vi "Calculate Odd Parity Bit (Array).vi"(0 "Bytes":u8[](array[numeric]) format="%02x", 11 "error in (no error)":errorcluster) -> (4 "Odd Parity Bit":u8, 15 "error out":errorcluster)   [LabVIEW 2018, in "MIPI RFFE API.lvlib"]
uses:
  MIPI RFFE API.lvlib
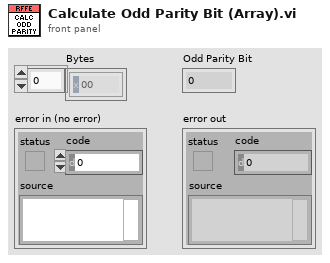
[diagram p1: front panel]
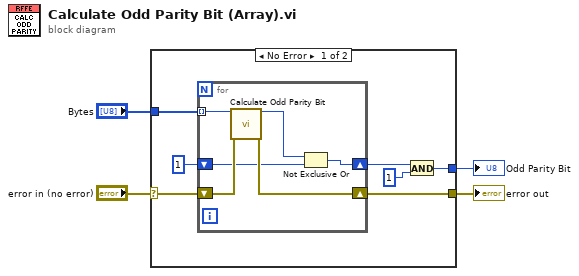
[diagram p0: block diagram]
diagram:
  n1 = case shown="No Error" "error in (no error)" {
    selector: "error in (no error)" -> [w11 w18]
    tunnel: [w10 w18] -> w3
    tunnel: "Bytes" -> [w9 _]
    tunnel: [w6 _] -> w1
    frame No Error {
      n2 = for {
        shift-right: [w16] -> w10
        shift-left: w11 -> [w17]
        tunnel: w9 -> [w15] mode=indexing
        shift-right: [w12] -> w7
        shift-left: u8 1 ("y") -> [w13]
        n3 = call "Calculate Odd Parity Bit.vi"("Byte"=w15, "error in (no error)"=w17) -> ("Odd Parity Bit"=w14:u8, "error out"=w16:errorcluster)  [unwired: 12 in]
        n4 = Not Exclusive Or(1:w13, 2:w14) -> (0:w12:u8)
      }
      n5 = And(x=w7, y=u8 1) -> (x .and. y?=w6:u8)
    }
    frame Error {
    }
  }
  "error out" <- w3
  "Odd Parity Bit" <- w1
